vi "get_LM_states.vi"(8 "error in (no error)":errorcluster caption="错误输入（无错误）", 11 "MotorSystem 输入":refnum<class "MotorSystem.lvclass">) -> (0 "error out":errorcluster caption="错误输出", 2 "LM states":cluster{"state -":bool, "state +":bool}[](array[cluster]), 3 "MotorSystem 输出":refnum<class "MotorSystem.lvclass">)   [LabVIEW 2016, in "MotionControl_UFO_3DOF.lvlib" / "MotorSystem.lvclass"]
uses:
  <userlib>/MotionControl_UFO_3DOF/MotorSystem/MotorSystem.lvclass
  <userlib>/MotionControl_UFO_3DOF/MotorSystem/MotorSystem.lvclass/MotorSystem.ctl
  <userlib>/MotionControl_UFO_3DOF/OneMotion/OneMotion.lvclass/OneMotion.ctl
  <userlib>/MotionControl_UFO_3DOF/LimitSwitch/LimitSwitch.lvclass/LimitSwitch.ctl
  <userlib>/UISimCanFunc_wrapper/VIs/sensor/Uim SFBK wrapper.vi
  <userlib>/MotionControl_UFO_3DOF/OneMotion/OneMotion.lvclass
  <userlib>/MotionControl_UFO_3DOF/LimitSwitch/LimitSwitch.lvclass
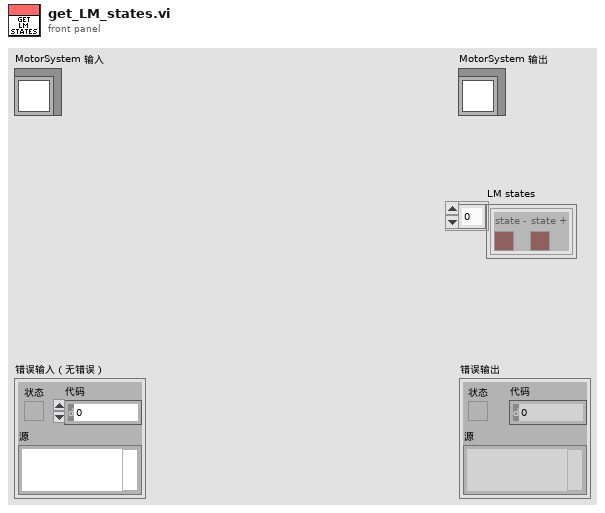
[diagram p1: front panel]
types:
  T1 = typedef "MotionControl_UFO_3DOF.lvlib/MotorSystem.lvclass/MotionCluster.ctl" = cluster{"OneMotion.lvclass":refnum<class "OneMotion.lvclass">, "connected?":bool, "default enabled?":bool, "enabled?":bool}
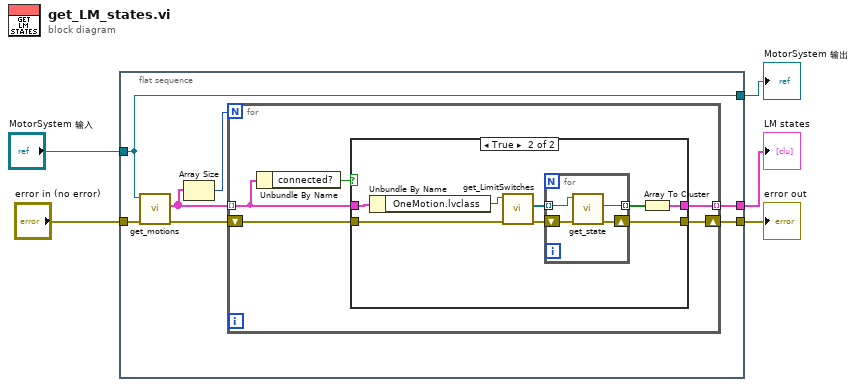
[diagram p0: block diagram]
diagram:
  n1 = flat-sequence {
    tunnel: [w7] -> w5
    tunnel: [w12] -> w3
    tunnel: "MotorSystem 输入" -> [w12]
    tunnel: "error in (no error)" -> [w9]
    tunnel: [w6] -> w1
    frame #0 {
      n2 = call <userlib>:"get_motions.vi"("error in (no error)"=w9, "MotorSystem输入"=w12) -> ("error out"=w8:errorcluster, "motions"=w10:T1[])  [unwired: 7 in, 1 out]
      n3 = Array Size(array=w10) -> (size(s)=w11:i32)
      n4 = for {
        N: w11 -> [_]
        tunnel: w10 -> [w14] mode=indexing
        shift-right: [w16] -> w7
        shift-left: w8 -> [w17]
        tunnel: [w15] -> w6 mode=indexing
        n5 = Unbundle By Name(w14) -> ("connected?"=w13:bool)
        n6 = case shown="True" w13 {
          tunnel: w14 -> [_ w26]
          tunnel: w17 -> [w18 w24]
          tunnel: [w18 w21] -> w16
          tunnel: [_ w19] -> w15
          frame False {
          }
          frame True {
            n7 = Unbundle By Name(w26) -> ("OneMotion.lvclass"=w25:refnum<class "OneMotion.lvclass">)
            n8 = call <userlib>:"get_LimitSwitches.vi"("error in (no error)"=w24, "OneMotion输入"=w25) -> ("error out"=w23:errorcluster, "LimitSwitches"=w22:refnum<class "LimitSwitch.lvclass">[])  [unwired: 7 in, 1 out]
            n9 = for {
              tunnel: [w30] -> w20 mode=indexing
              tunnel: w22 -> [w28] mode=indexing
              shift-right: [w27] -> w21
              shift-left: w23 -> [w29]
              n10 = call <userlib>:"get_state.vi"("error in (no error)"=w29, "LimitSwitch输入"=w28) -> ("error out"=w27:errorcluster, "state"=w30:bool)  [unwired: 7 in, 1 out]
            }
            n11 = Array To Cluster(array=w20) -> (cluster=w19:cluster{"[0]":bool, "[1]":bool})
          }
        }
      }
    }
  }
  "error out" <- w5
  "MotorSystem 输出" <- w3
  "LM states" <- w1
